vi "BRig_FPGA_v3,94__PortC.vi"() -> ()   [LabVIEW 2014]
uses:
  <vilib>/rvi/Emulation/niFpgaGetClockAttributes.vi
  <vilib>/rvi/Emulation/niFpgaSctlEmulationGetInTimedLoop.vi
  <vilib>/rvi/Emulation/niFpgaEmulationReportErrorSimple.vi
  <vilib>/rvi/eio/common/nirviEmuTemplateMethod_errors.vi
  <vilib>/rvi/Emulation/niFpgaCriticalErrorInLSC.vi
  <vilib>/eio/EIONode/EIONode.xnode
panel:
  in  "AnaOut1_Pair":u16
  in  "AnaOut0_Pair":u16
  out "fpga_solenoid_R":bool
  out "fpga_solenoid_L":bool
  out "fpga_laser2":bool
  out "fpga_laser1":bool
  in  "L2Led_ON":bool
  in  "L1Led_ON":bool
  in  "Rising(F)_or_Falling(T)":bool
  in  "Solenoid_trig_R":bool
  in  "Solenoid_trig_L":bool
  in  "Solenoid_nTotal_R":u32=100
  in  "Solenoid_nTotal_L":u32=100
  in  "L2Led_Baseline":bool
  in  "L1Led_Baseline":bool
  in  "CueLed_Baseline":bool
  in  "I_allReward":bool
  in  "AnaOut_1":i16
  in  "CueLed_Event":bool
  in  "CueLed_nValley":u32=100
  in  "CueLed_nPeak":u32=100
  in  "LC_Event_l2":bool
  in  "LC_Laser_l2":bool
  in  "LC_nShutter_l2":u32=100
  in  "LC_nValley_l2":u32=100
  in  "LC_nPeak_l2":u32=100
  in  "LR_wrong_nDelay_l2":u32
  in  "LR_reward_nDelay_l2":u32
  in  "LR_wrong_nTotal_l2":u32=100
  in  "LR_reward_nTotal_l2":u32=100
  in  "LR_wrong_laser_l2":bool
  in  "LR_wrong_Event_l2":bool
  in  "LR_reward_Laser_l2":bool
  in  "LR_reward_Event_l2":bool
  out "AnaIn_1":i16
  out "AnaIn_0":i16
  out "timeTrial_count":u32
  in  "timeTrial_trig":bool
  in  "k1__counter_per_ms":u16=100 min=100 max=40000 step=1
  in  "LC_nShutter_l1":u32=100
  in  "AnaOut_0":i16
  in  "LC_nValley_l1":u32=100
  in  "LC_nPeak_l1":u32=100
  in  "LC_Event_l1":bool
  in  "LR_wrong_nTotal_l1":u32=100
  in  "LR_wrong_nDelay_l1":u32
  in  "LR_reward_nTotal_l1":u32=100
  in  "LR_reward_nDelay_l1":u32
  in  "LR_reward_Event_l1":bool
  in  "LR_wrong_Event_l1":bool
  out "SelectWrong":bool
  out "SelectReward":bool
  in  "LR_wrong_Laser_l1":bool
  in  "LR_reward_Laser_l1":bool
  in  "Left(F)_or_Right(T)":bool
  in  "ignoreWrong":bool
  in  "SelectionState":bool
  in  "LC_Laser_l1":bool
  in  "FPGA_Stop":bool
  in  "audioTrigger_L":bool
  in  "audioTrigger_R":bool
  in  "audioFreq_L_kHz":u8=14 min=1 max=14 step=1
  in  "audioAmp_L":u16=1 min=1 max=32767 step=1
  in  "audioFreq_R_kHz":u8=14 min=1 max=14 step=1
  in  "audioAmp_R":u16=1 min=1 max=32767 step=1
  in  "A3_SL":bool
  in  "A1_SR":bool
  in  "Counts_Reset":bool
  out "A4_LickR":u32
  out "A2_LickL":u32
  in  "A6_Act":bool
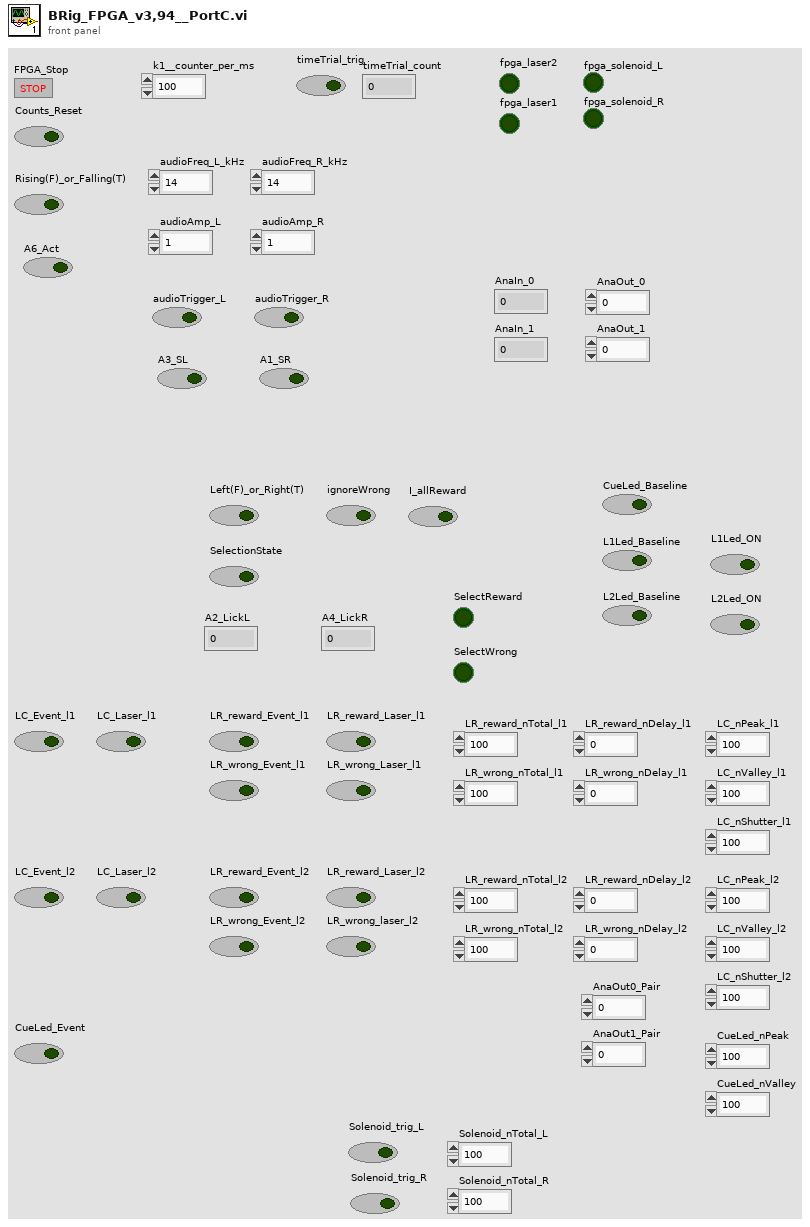
[diagram p1: front panel]
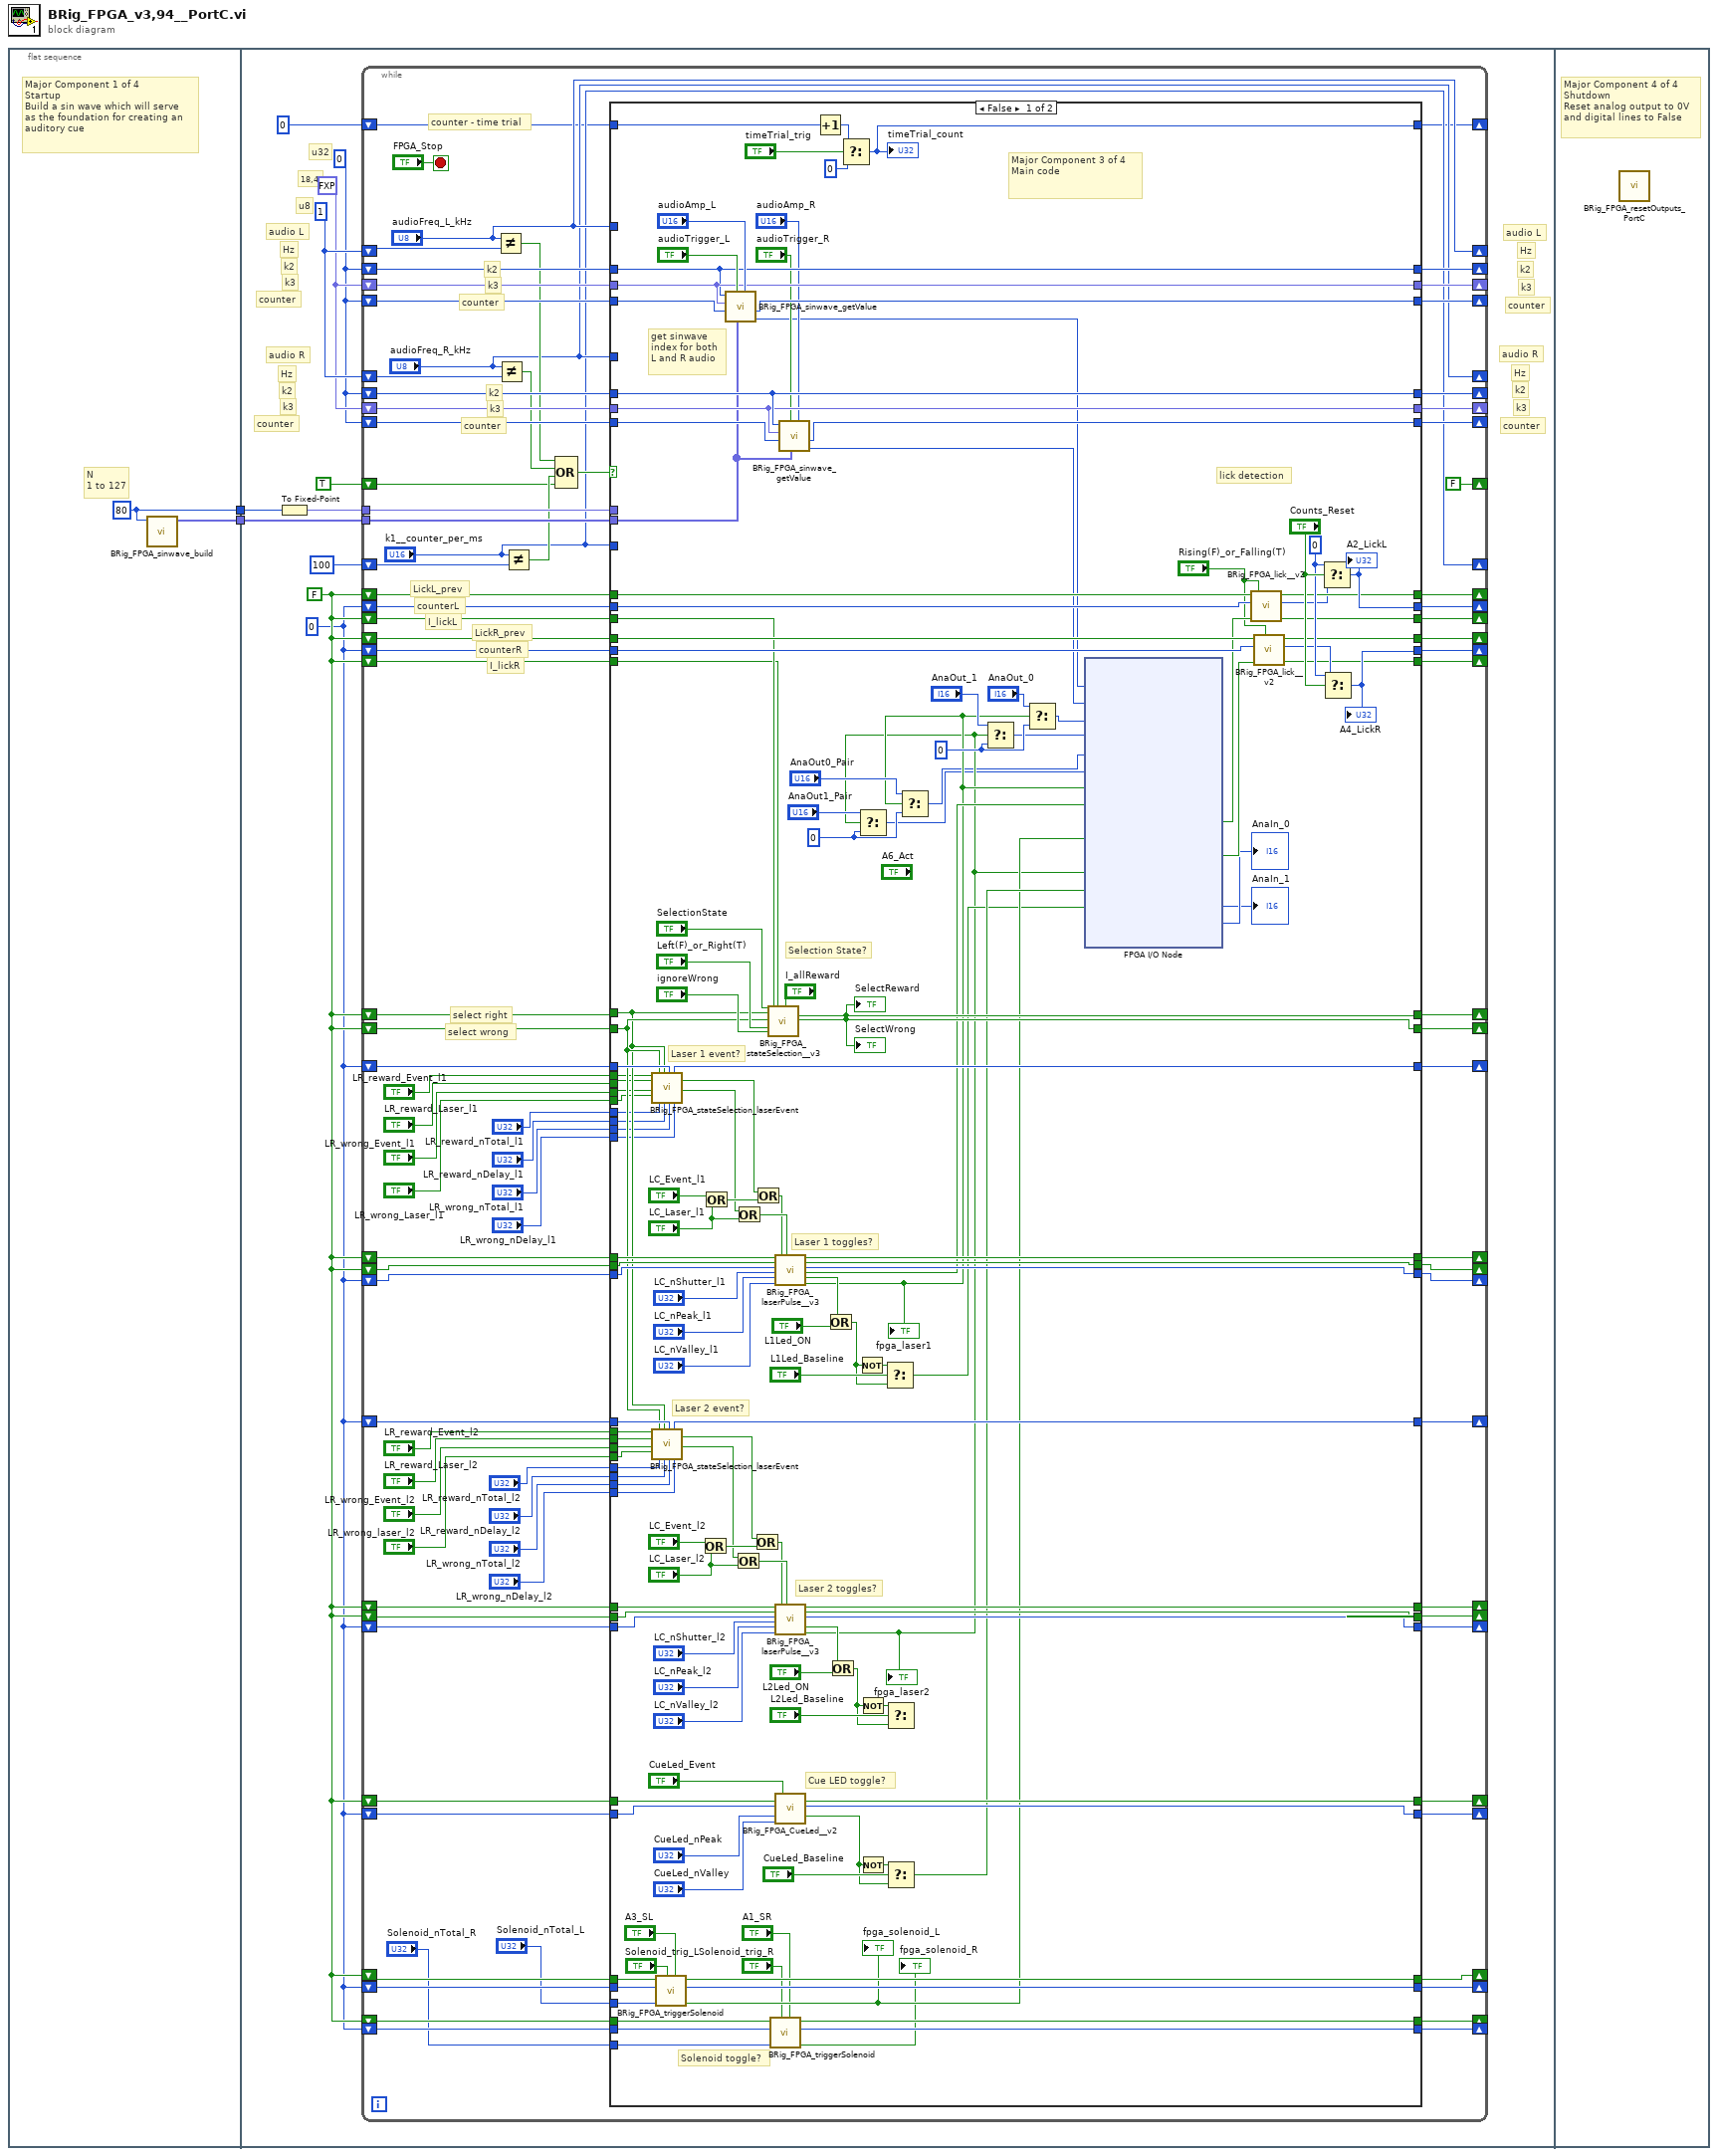
[diagram p0: block diagram]
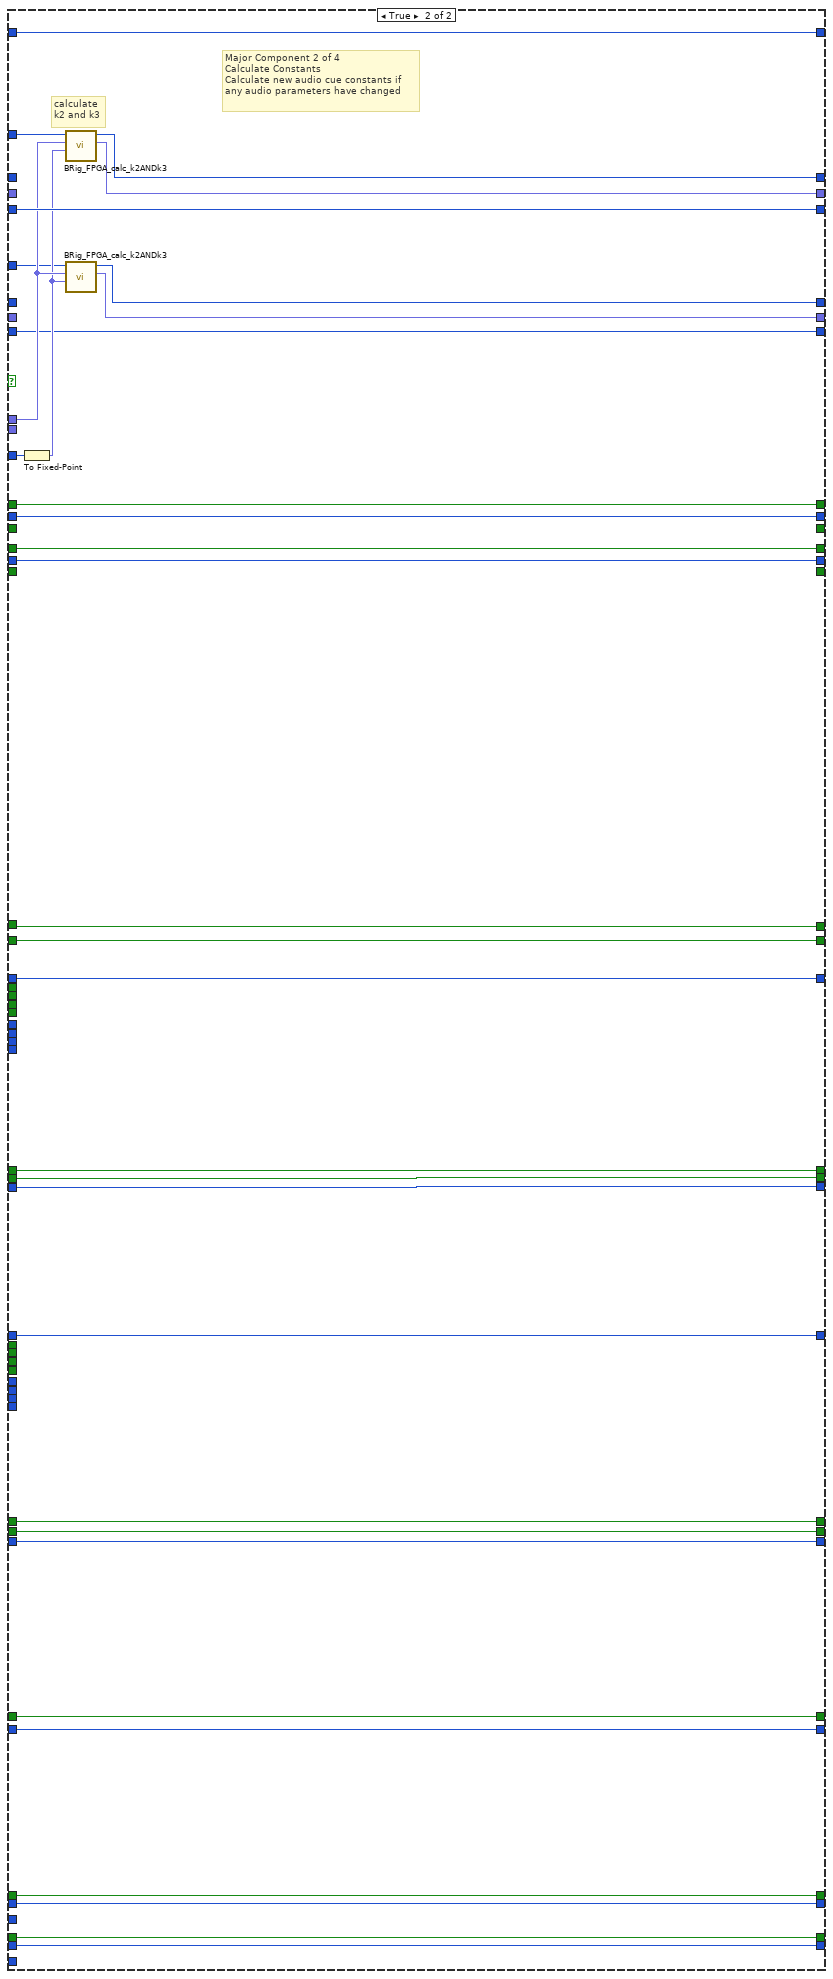
[diagram p2: hidden frame]
diagram:
  n1 = flat-sequence {
    tunnel: [w4] -> w2
    tunnel: [w3] -> w1
    tunnel: w2 -> [w15]
    tunnel: w1 -> [w14]
    frame #0 {
      w3 = 80 ("dimension size")
      # "Major Component 1 of 4\nStartup\nBuild a sin wave which will serve\nas the foundation for creating an\nauditory cue"
      # "N\n1 to 127"
      n2 = call "BRig_FPGA_sinwave_build.vi"("input_Npts"=w3) -> ("output_array_sin"=w4:fxp<+/-,16,2>[])  [unwired: 10 in]
    }
    frame #1 {
      w5 = u32 0
      w6 = FALSE
      w10 = u32 0
      w11 = fxp<+,18,4> 0.0
      w12 = u8 1
      # "counter"
      # "k3"
      # "k2"
      # "counter"
      # "k3"
      # "k2"
      # "counter"
      # "counter"
      # "u32"
      # "k3"
      # "k2"
      # "k3"
      # "18,4"
      # "u8"
      # "Hz"
      # "Hz"
      # "audio R"
      # "audio L"
      # "Hz"
      # "k2"
      # "Hz"
      # "audio R"
      # "audio L"
      n3 = To Fixed-Point(number=w14) -> (fixed-point=w13:fxp<+,7,7>)  [unwired: 1 in]
      n4 = while {
        shift-right: ["audioFreq_L_kHz"] -> _
        shift-left: w12 -> [w106]
        shift-right: [w100] -> _
        shift-left: w10 -> [w104]
        shift-right: ["audioFreq_R_kHz"] -> _
        shift-left: w12 -> [w96]
        tunnel: w15 -> [w103]
        tunnel: w13 -> [w102]
        shift-right: [w99] -> _
        shift-left: w11 -> [w101]
        shift-right: [w97] -> _
        shift-left: w10 -> [w98]
        shift-right: [w94] -> _
        shift-left: w10 -> [w95]
        shift-right: [w92] -> _
        shift-left: w11 -> [w93]
        shift-right: [w90] -> _
        shift-left: w10 -> [w91]
        shift-right: ["k1__counter_per_ms"] -> _
        shift-left: u16 100 ("y") -> [w89]
        shift-right: [FALSE] -> _
        shift-left: TRUE -> [w84]
        shift-right: [w77] -> _
        shift-left: w6 -> [w79]
        shift-right: [w76] -> _
        shift-left: w6 -> [w78]
        shift-right: [w74] -> _
        shift-left: w5 -> [w75]
        shift-right: [w72] -> _
        shift-left: w5 -> [w73]
        shift-right: [w69] -> _
        shift-left: w6 -> [w71]
        shift-right: [w68] -> _
        shift-left: w6 -> [w70]
        shift-right: [w66] -> _
        shift-left: w6 -> [w67]
        shift-right: [w64] -> _
        shift-left: w6 -> [w65]
        shift-right: [w62] -> _
        shift-left: u32 0 -> [w63]
        shift-right: [w60] -> _
        shift-left: w5 -> [w61]
        shift-right: [w59] -> _
        shift-left: w6 -> [w56]
        shift-right: [w58] -> _
        shift-left: w6 -> [w55]
        shift-right: [w57] -> _
        shift-left: w5 -> [w54]
        shift-right: [w52] -> _
        shift-left: w5 -> [w53]
        shift-right: [w51] -> _
        shift-left: w6 -> [w48]
        shift-right: [w50] -> _
        shift-left: w6 -> [w47]
        shift-right: [w49] -> _
        shift-left: w5 -> [w46]
        shift-right: [w45] -> _
        shift-left: w6 -> [w43]
        shift-right: [w44] -> _
        shift-left: w5 -> [w42]
        shift-right: [w24] -> _
        shift-left: w5 -> [w25]
        shift-right: [w21] -> _
        shift-left: w6 -> [w23]
        shift-right: [w18] -> _
        shift-left: w6 -> [w20]
        shift-right: [w17] -> _
        shift-left: w5 -> [w19]
        stop <- "FPGA_Stop" stop-if-true
        # "counter"
        # "k3"
        # "k2"
        # "counter"
        # "k3"
        # "k2"
        # "counter - time trial"
        # "I_lickR"
        # "counterR"
        # "LickR_prev"
        # "I_lickL"
        # "counterL"
        # "LickL_prev"
        # "select wrong"
        # "select right"
        n5 = Not Equal?(x="audioFreq_L_kHz", y=w106) -> (x != y?=w88:bool)
        n6 = Not Equal?(x="audioFreq_R_kHz", y=w96) -> (x != y?=w87:bool)
        n7 = Not Equal?(x="k1__counter_per_ms", y=w89) -> (x != y?=w85:bool)
        n8 = Compound Arithmetic op=OR(w88, w87, w85, w84) -> (w86:bool)
        n9 = case shown="False" w86 {
          tunnel: w104 -> [w243 _]
          tunnel: "audioFreq_L_kHz" -> [_ w289]
          tunnel: w103 -> [w236 _]
          tunnel: w102 -> [_ w285]
          tunnel: "k1__counter_per_ms" -> [_ w290]
          tunnel: w101 -> [w244 _]
          tunnel: [w243 w288] -> w100
          tunnel: [w244 w287] -> w99
          tunnel: w98 -> [w248 w286]
          tunnel: [w245 w286] -> w97
          tunnel: w95 -> [w240 _]
          tunnel: [w240 w281] -> w94
          tunnel: w93 -> [w239 _]
          tunnel: [w239 w282] -> w92
          tunnel: w91 -> [w242 w280]
          tunnel: "audioFreq_R_kHz" -> [_ w283]
          tunnel: [w241 w280] -> w90
          tunnel: w79 -> [w231 w279]
          tunnel: w78 -> [w230 w278]
          tunnel: [w235 w279] -> w77
          tunnel: [w228 w278] -> w76
          tunnel: w75 -> [w232 w277]
          tunnel: [w258 w277] -> w74
          tunnel: w73 -> [w229 w276]
          tunnel: [w255 w276] -> w72
          tunnel: w71 -> [w182 w275]
          tunnel: w70 -> [w183 w274]
          tunnel: [w202 w275] -> w69
          tunnel: [w251 w274] -> w68
          tunnel: [w221 w271] -> w59
          tunnel: [w222 w270] -> w58
          tunnel: [w223 w269] -> w57
          tunnel: w67 -> [w225 _]
          tunnel: [w234 _] -> w66
          tunnel: w65 -> [w224 _]
          tunnel: [w226 _] -> w64
          tunnel: w63 -> [w213 w273]
          tunnel: [w210 w273] -> w62
          tunnel: w61 -> [w201 w272]
          tunnel: [w200 w272] -> w60
          tunnel: w56 -> [w199 w271]
          tunnel: w55 -> [w198 w270]
          tunnel: w54 -> [w197 w269]
          tunnel: w53 -> [w185 w268]
          tunnel: [w184 w268] -> w52
          tunnel: [w180 w267] -> w51
          tunnel: [w179 w266] -> w50
          tunnel: [w178 w265] -> w49
          tunnel: w48 -> [w177 w267]
          tunnel: w47 -> [w176 w266]
          tunnel: w46 -> [w175 w265]
          tunnel: [w172 w264] -> w45
          tunnel: [w171 w263] -> w44
          tunnel: w43 -> [w170 w264]
          tunnel: w42 -> [w169 w263]
          tunnel: "LR_reward_Event_l1" -> [w154 _]
          tunnel: "LR_reward_Laser_l1" -> [w153 _]
          tunnel: "LR_wrong_Event_l1" -> [w152 _]
          tunnel: "LR_wrong_Laser_l1" -> [w151 _]
          tunnel: "LR_reward_nTotal_l1" -> [w150 _]
          tunnel: "LR_reward_nDelay_l1" -> [w149 _]
          tunnel: "LR_wrong_nTotal_l1" -> [w148 _]
          tunnel: "LR_wrong_nDelay_l1" -> [w147 _]
          tunnel: "LR_reward_Event_l2" -> [w146 _]
          tunnel: "LR_reward_Laser_l2" -> [w145 _]
          tunnel: "LR_wrong_Event_l2" -> [w144 _]
          tunnel: "LR_wrong_laser_l2" -> [w143 _]
          tunnel: "LR_reward_nTotal_l2" -> [w142 _]
          tunnel: "LR_reward_nDelay_l2" -> [w141 _]
          tunnel: "LR_wrong_nTotal_l2" -> [w140 _]
          tunnel: "LR_wrong_nDelay_l2" -> [w139 _]
          tunnel: w25 -> [w138 w262]
          tunnel: [w133 w262] -> w24
          tunnel: w23 -> [w137 w261]
          tunnel: "Solenoid_nTotal_L" -> [w136 _]
          tunnel: [w132 w261] -> w21
          tunnel: w20 -> [w128 w260]
          tunnel: w19 -> [w127 w259]
          tunnel: [w126 w260] -> w18
          tunnel: [w125 w259] -> w17
          tunnel: "Solenoid_nTotal_R" -> [w124 _]
          frame False {
            w112 = u16 0 ("f")
            w166 = i16 0 ("f")
            w256 = u32 0 ("t")
            # "Solenoid toggle?"
            # "Cue LED toggle?"
            # "Laser 2 toggles?"
            # "Laser 2 event?"
            # "Laser 1 toggles?"
            # "Selection State?"
            # "Laser 1 event?"
            # "Major Component 3 of 4\nMain code"
            # "get sinwave\nindex for both\nL and R audio"
            # "lick detection"
            n10 = call "BRig_FPGA_stateSelection_laserEvent.vi"("I_LR_reward"=w154, "I_LR_reward_laser"=w153, "I_LR_wrong"=w152, "I_LR_wrong_laser"=w151, "I_selectWrong"=w183, "laser_reward_nTotal"=w150, "I_selectReward"=w182, "laser_reward_nDelay"=w149, "counter"=w201, "laser_wrong_nTotal"=w148, "laser_wrong_nDelay"=w147) -> ("output_counter"=w200:u32, "output_I_laserEvent"=w196:bool, "output_I_laserOn"=w195:bool)  [unwired: 6 in]
            n11 = call "BRig_FPGA_stateSelection_laserEvent.vi"("I_LR_reward"=w146, "I_LR_reward_laser"=w145, "I_LR_wrong"=w144, "I_LR_wrong_laser"=w143, "I_selectWrong"=w183, "laser_reward_nTotal"=w142, "I_selectReward"=w182, "laser_reward_nDelay"=w141, "counter"=w185, "laser_wrong_nTotal"=w140, "laser_wrong_nDelay"=w139) -> ("output_counter"=w184:u32, "output_I_laserEvent"=w181:bool, "output_I_laserOn"=w186:bool)  [unwired: 6 in]
            n12 = call "BRig_FPGA_triggerSolenoid.vi"("input_Solenoid_MTrig"="A3_SL", "input_Solenoid_trig"="Solenoid_trig_L", "input_threshold"=w136, "input_counter"=w138, "input_trig"=w137) -> ("output_Solenoid_OnOff"=w131:bool, "output_counter"=w133:u32, "output_trig"=w132:bool)  [unwired: 4 in]
            "fpga_solenoid_L" <- w131
            n13 = Or(x="LC_Event_l2", y="LC_Laser_l2") -> (x .or. y?=w190:bool)
            n14 = Or(x="LC_Event_l1", y="LC_Laser_l1") -> (x .or. y?=w217:bool)
            n15 = call "BRig_FPGA_sinwave_getValue.vi"("audioAmp"="audioAmp_L", "sinwave"=w236, "audioTrigger"="audioTrigger_L", "counter"=w248, "k3"=w244, "k2"=w243) -> ("output_audioValue"=w208:i16, "output_counter"=w245:u32)  [unwired: 4 in]
            n16 = Or(x=w186, y="LC_Laser_l2") -> (x .or. y?=w188:bool)
            n17 = Or(x=w195, y="LC_Laser_l1") -> (x .or. y?=w215:bool)
            n18 = Or(x=w181, y=w190) -> (x .or. y?=w187:bool)
            n19 = Or(x=w196, y=w217) -> (x .or. y?=w214:bool)
            n20 = call "BRig_FPGA_stateSelection__v3.vi"("I_selectionState"="SelectionState", "I_selectRight"=w182, "I_selectWrong"=w183, "I_Left(F)_or_Right(T)"="Left(F)_or_Right(T)", "I_ignoreWrong"="ignoreWrong", "I_lickL"=w225, "I_lickR"=w224, "I_allReward"="I_allReward") -> ("output__I_selectRight"=w202:bool, "output__I_selectWrong"=w251:bool)  [unwired: 18 in]
            "SelectWrong" <- w251
            "SelectReward" <- w202
            n21 = call "BRig_FPGA_triggerSolenoid.vi"("input_Solenoid_MTrig"="A1_SR", "input_Solenoid_trig"="Solenoid_trig_R", "input_threshold"=w124, "input_counter"=w127, "input_trig"=w128) -> ("output_Solenoid_OnOff"=→"fpga_solenoid_R":bool, "output_counter"=w125:u32, "output_trig"=w126:bool)  [unwired: 4 in]
            n22 = call "BRig_FPGA_laserPulse__v3.vi"("I_shutter"=w199, "I_peak"=w198, "count"=w197, "laser_Nshutter"="LC_nShutter_l1", "laser_Npeak"="LC_nPeak_l1", "laser_Nvalley"="LC_nValley_l1", "I_laserEvent"=w214, "I_laser"=w215) -> ("output_I_shutter"=w221:bool, "output_I_peak"=w222:bool, "output_count"=w223:u32, "output_shutter"=w115:bool, "output_led"=w120:bool, "output_laser"=w110:bool)  [unwired: 6 in]
            "fpga_laser1" <- w110
            n23 = call "BRig_FPGA_laserPulse__v3.vi"("I_shutter"=w177, "I_peak"=w176, "count"=w175, "laser_Nshutter"="LC_nShutter_l2", "laser_Npeak"="LC_nPeak_l2", "laser_Nvalley"="LC_nValley_l2", "I_laserEvent"=w187, "I_laser"=w188) -> ("output_I_shutter"=w180:bool, "output_I_peak"=w179:bool, "output_count"=w178:u32, "output_led"=w117:bool, "output_laser"=w109:bool)  [unwired: 6 in, 1 out]
            "fpga_laser2" <- w109
            n24 = call "BRig_FPGA_CueLed__v2.vi"("I_peak"=w170, "count"=w169, "laser_Npeak"="CueLed_nPeak", "laser_Nvalley"="CueLed_nValley", "I_CueLed_Event"="CueLed_Event") -> ("output_I_peak"=w172:bool, "output_count"=w171:u32, "output_led"=w159:bool)  [unwired: 12 in]
            n25 = call "BRig_FPGA_sinwave_getValue.vi"("audioAmp"="audioAmp_R", "sinwave"=w236, "audioTrigger"="audioTrigger_R", "counter"=w242, "k3"=w239, "k2"=w240) -> ("output_audioValue"=w207:i16, "output_counter"=w241:u32)  [unwired: 4 in]
            n26 = Increment(x=w213) -> (x+1=w212:u32)
            n27 = Or(x=w120, y="L1Led_ON") -> (x .or. y?=w119:bool)
            n28 = Or(x=w117, y="L2Led_ON") -> (x .or. y?=w116:bool)
            n29 = Select(t=w212, s="timeTrial_trig", f=u32 0) -> (s? t:f=w210:u32)
            "timeTrial_count" <- w210
            n30 = Not(x=w119) -> (.not. x?=w158:bool)
            n31 = Select(t="AnaOut1_Pair", s=w109, f=w112) -> (s? t:f=w108:u16)
            n32 = Not(x=w116) -> (.not. x?=w156:bool)
            n33 = Not(x=w159) -> (.not. x?=w161:bool)
            n34 = Select(t=w158, s="L1Led_Baseline", f=w119) -> (s? t:f=w122:bool)
            n35 = Select(t=w156, s="L2Led_Baseline", f=w116) -> ()  [unwired: 1 out]
            n36 = Select(t=w161, s="CueLed_Baseline", f=w159) -> (s? t:f=w162:bool)
            n37 = Select(t="AnaOut0_Pair", s=w110, f=w112) -> (s? t:f=w107:u16)
            n38 = Select(t="AnaOut_1", s=w109, f=w166) -> (s? t:f=w164:i16)
            n39 = Select(t="AnaOut_0", s=w110, f=w166) -> (s? t:f=w167:i16)
            n40 = xnode "FPGA I/O Node"("AudioOut/Left"=w208, "AudioOut/Right"=w207, "ConnectorC/AO0"=w167, "ConnectorC/AO1"=w164, "ConnectorB/AO0"=w107, "ConnectorB/AO1"=w108, "ConnectorC/DIO0"=w110, "ConnectorC/DIO1"=w115, "ConnectorC/DIO3"=w131, "ConnectorC/DIO5"=w109, "ConnectorC/DIO6"=w162, "ConnectorC/DIO7"=w122) -> ("ConnectorC/DIO2"=w206:bool, "ConnectorC/DIO4"=w205:bool, "ConnectorC/AI0"=→"AnaIn_0":i16, "ConnectorC/AI1"=→"AnaIn_1":i16)  [unwired: 16 in, 16 out]
            n41 = call "BRig_FPGA_lick__v2.vi"("Rising(F)_or_Falling(T)"="Rising(F)_or_Falling(T)", "I_stateDetector_new"=w206, "counter"=w232, "I_stateDetector_prev"=w231) -> ("output_I_lick"=w234:bool, "output_counter"=w233:u32, "output_I_stateDetector_prev"=w235:bool)  [unwired: 5 in]
            n42 = call "BRig_FPGA_lick__v2.vi"("Rising(F)_or_Falling(T)"="Rising(F)_or_Falling(T)", "I_stateDetector_new"=w205, "counter"=w229, "I_stateDetector_prev"=w230) -> ("output_I_lick"=w226:bool, "output_counter"=w227:u32, "output_I_stateDetector_prev"=w228:bool)  [unwired: 5 in]
            n43 = Select(t=w256, s="Counts_Reset", f=w233) -> (s? t:f=w258:u32)
            "A2_LickL" <- w258
            n44 = Select(t=w256, s="Counts_Reset", f=w227) -> (s? t:f=w255:u32)
            "A4_LickR" <- w255
          }
          frame True {
            # "Major Component 2 of 4\nCalculate Constants\nCalculate new audio cue constants if\nany audio parameters have changed"
            # "calculate\nk2 and k3"
            n45 = To Fixed-Point(number=w290) -> (fixed-point=w284:fxp<+,16,16>)  [unwired: 1 in]
            n46 = call "BRig_FPGA_calc_k2ANDk3.vi"("input_k1[count/ms]"=w284, "input_Npts"=w285, "input_freq[kHz]"=w289) -> ("output_k3"=w287:fxp<+,18,4>, "output_k2"=w288:u32)  [unwired: 7 in]
            n47 = call "BRig_FPGA_calc_k2ANDk3.vi"("input_k1[count/ms]"=w284, "input_Npts"=w285, "input_freq[kHz]"=w283) -> ("output_k3"=w282:fxp<+,18,4>, "output_k2"=w281:u32)  [unwired: 7 in]
          }
        }
      }
    }
    frame #2 {
      # "Major Component 4 of 4\nShutdown\nReset analog output to 0V\nand digital lines to False"
      n48 = call "BRig_FPGA_resetOutputs_PortC.vi"() -> ()  [unwired: 12 in]
    }
  }
